vi "KepcoDCPwr Error-Query.vi"(0 "VISA Session":refnum<visa-resource-name>, 5 "Model In":string, 7 "channel name (\"\")":string="\"\"", 11 "error in (no error)":errorcluster {"code" format="%.0x"}) -> (4 "VISA Session Out":refnum<visa-resource-name>, 6 "Model Out":string, 8 "channel name out (\"\")":string="\"\"" caption="channel name Out (\"\")", 10 "error code":i32, 14 "error message":string, 15 "error out":errorcluster {"code" format="%.0x"})   [LabVIEW 2013]
doc: "This VI reads an error code and a message from the instrument's error queue."
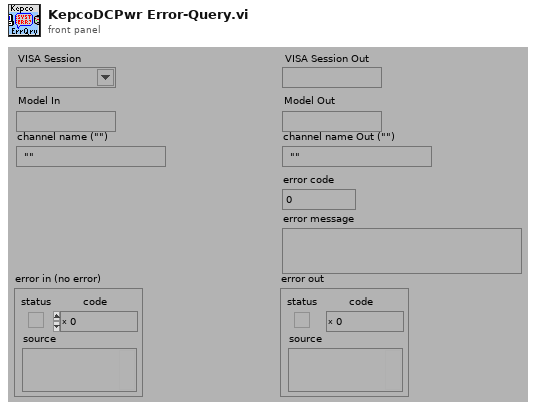
[diagram p1: front panel]
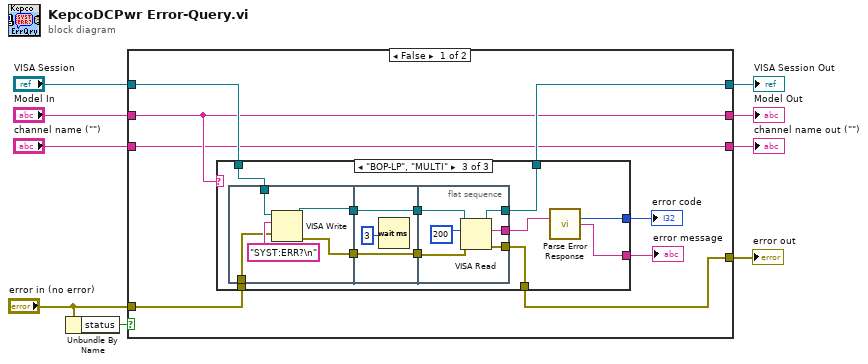
[diagram p0: block diagram]
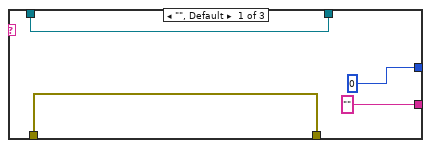
[diagram p2: hidden frame]
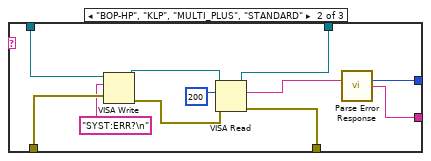
[diagram p3: hidden frame]
diagram:
  n1 = Unbundle By Name("error in (no error)") -> ("status"=w1:bool)
  n2 = case shown="False" w1 {
    tunnel: "VISA Session" -> [w17 w61]
    tunnel: [w16 w61] -> w8
    tunnel: [w15 w60] -> w7
    tunnel: "error in (no error)" -> [w14 w60]
    tunnel: "Model In" -> [w13 w59]
    tunnel: [w13 w59] -> w5
    tunnel: "channel name (\"\")" -> [w12 w58]
    tunnel: [w12 w58] -> w3
    frame False {
      n3 = case shown="\"BOP-LP\", \"MULTI\"" w13 {
        tunnel: [w19 w25 w34] -> w16
        tunnel: w17 -> [w19 w32 w43]
        tunnel: w14 -> [w21 w31 w42]
        tunnel: [w21 w26 w35] -> w15
        tunnel: [0 w30 w41] -> w11
        tunnel: ["" w29 w40] -> w10
        frame "", Default {
        }
        frame "BOP-HP", "KLP", "MULTI_PLUS", "STANDARD" {
          n4 = VISA Write(VISA resource name=w32, write buffer="SYST:ERR?\n", error in (no error)=w31) -> (VISA resource name out=w27:refnum<visa-resource-name>, error out=w28:errorcluster)  [unwired: 1 out]
          n5 = VISA Read(VISA resource name=w27, byte count=u32 200 ("byte count (0)"), error in (no error)=w28) -> (VISA resource name out=w25:refnum<visa-resource-name>, read buffer=w24:string, error out=w26:errorcluster)  [unwired: 1 out]
          n6 = call "Parse Error Response.vi"("Error String"=w24) -> ("error code"=w30:i32, "error message"=w29:string)  [unwired: 13 out]
        }
        frame "BOP-LP", "MULTI" {
          n7 = flat-sequence {
            tunnel: w43 -> [w47]
            tunnel: w42 -> [w46]
            tunnel: [w45] -> w39
            tunnel: [w44] -> w38
            tunnel: w39 -> [w51]
            tunnel: w38 -> [w50]
            tunnel: [w51] -> w37
            tunnel: [w50] -> w36
            tunnel: [w53] -> w34
            tunnel: w37 -> [w54]
            tunnel: w36 -> [w52]
            tunnel: [w56] -> w35
            tunnel: [w55] -> w33
            frame #0 {
              n8 = VISA Write(VISA resource name=w47, write buffer="SYST:ERR?\n", error in (no error)=w46) -> (VISA resource name out=w44:refnum<visa-resource-name>, error out=w45:errorcluster)  [unwired: 1 out]
            }
            frame #1 {
              n9 = Wait (ms)(milliseconds to wait=3) -> ()  [unwired: 1 out]
            }
            frame #2 {
              n10 = VISA Read(VISA resource name=w52, byte count=u32 200 ("byte count (0)"), error in (no error)=w54) -> (VISA resource name out=w53:refnum<visa-resource-name>, read buffer=w55:string, error out=w56:errorcluster)  [unwired: 1 out]
            }
          }
          n11 = call "Parse Error Response.vi"("Error String"=w33) -> ("error code"=w41:i32, "error message"=w40:string)  [unwired: 13 out]
        }
      }
      "error code" <- w11
      "error message" <- w10
    }
    frame True {
    }
  }
  "error out" <- w7
  "VISA Session Out" <- w8
  "Model Out" <- w5
  "channel name out (\"\")" <- w3
